vi "FitLinear (SubVI).vi"(0 "Normalized Intensity vs Radius in":cluster{dbl[], dbl[]}, 1 "x values":dbl[](array[numeric]), 2 "y values":dbl[](array[numeric]), 3 "Estimated mean":dbl, 4 "Estimated width":dbl, 6 "parameter bounds":T1={"slope min"=-inf, "slope max"=inf, "intercept min"=-inf, "intercept max"=inf}, 7 "Nsigma Low":dbl=4.0 format="%#_13g", 8 "Use all points":bool, 9 "Nsigma High":dbl=4.0 format="%#_13g") -> (14 "data plot":cluster{dbl[], dbl[]}(graph), 15 "derivative data plot with linear fit":T2(graph), 16 "slope":dbl, 17 "intercept":dbl, 18 "error":i32, 19 "residue":dbl)   [LabVIEW 2016]
uses:
  <vilib>/Analysis/NI_AALPro.lvlib
panel:
  # "RESULTS"
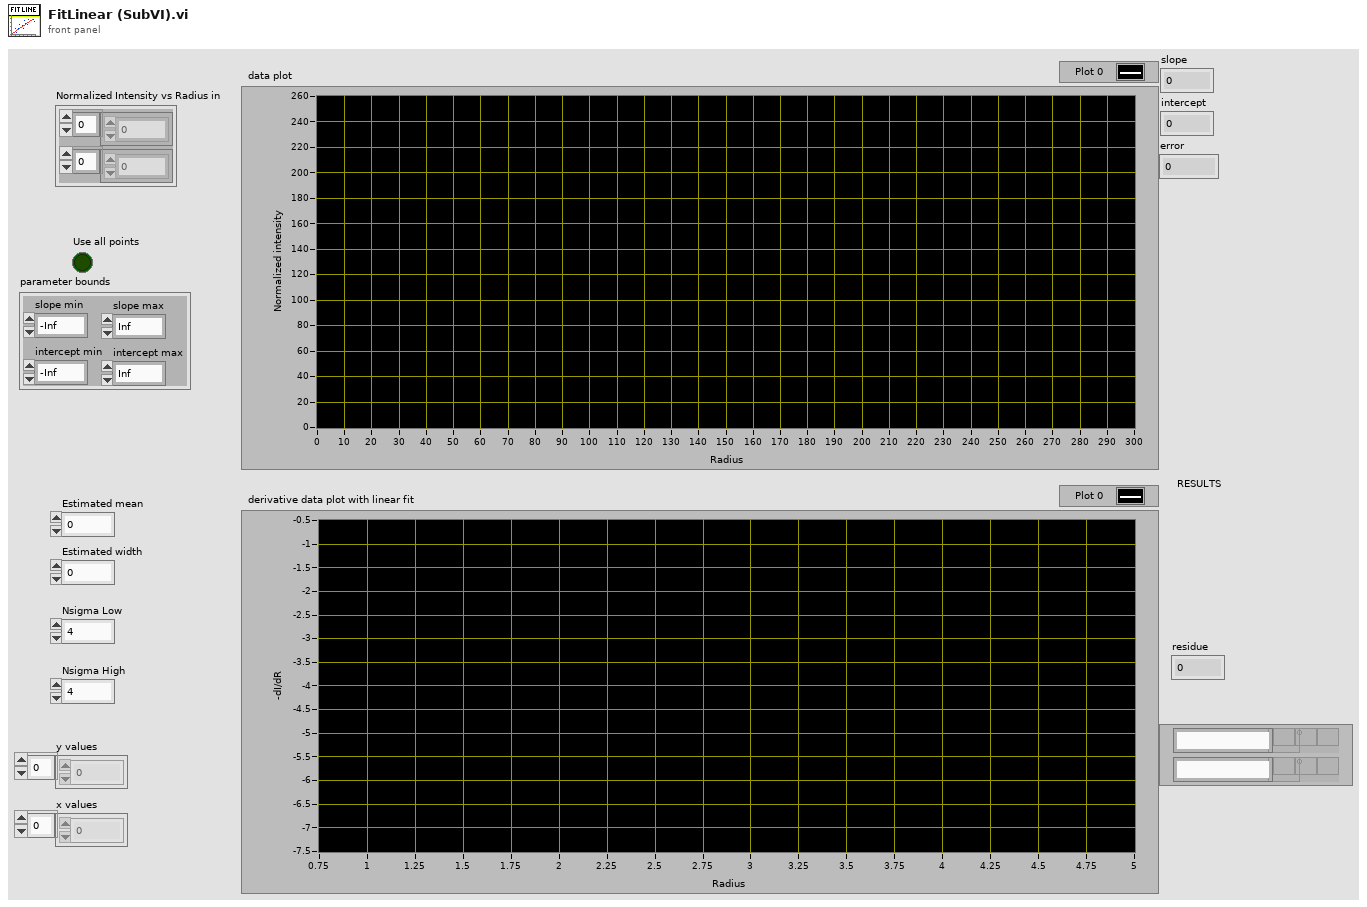
[diagram p1: front panel]
types:
  T1 = cluster{"slope min":dbl, "slope max":dbl, "intercept min":dbl, "intercept max":dbl}
  T2 = cluster{"Radius bins":dbl[], "Best Gaussian Fit":dbl[]}[]
  T3 = cluster{"x values":dbl[], "Best Linear Fit":dbl[]}
  T4 = cluster{"x values":dbl[], "Best Linear Fit":dbl[]}[]
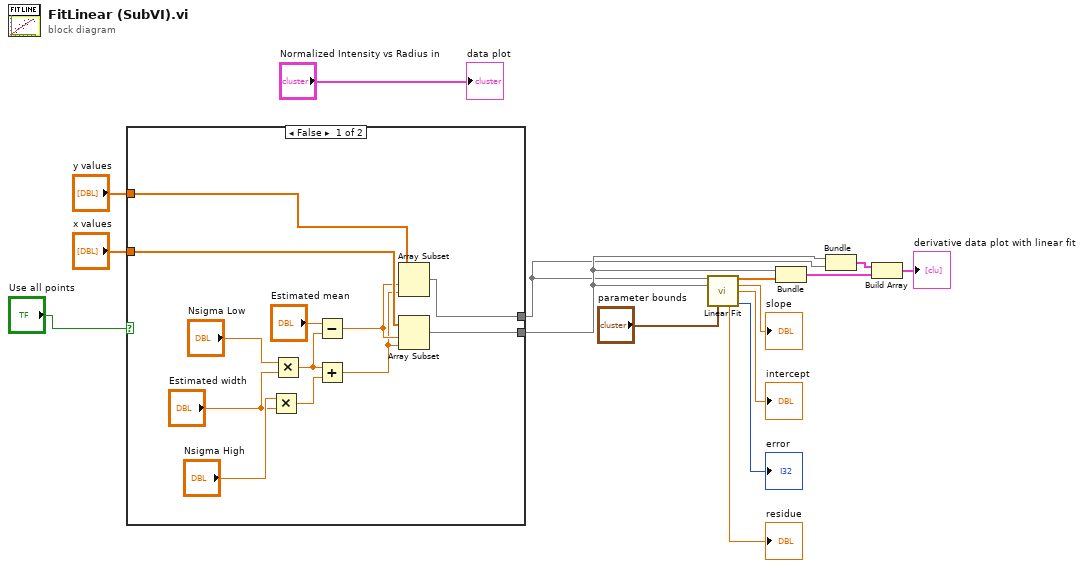
[diagram p0: block diagram]
diagram:
  n1 = case shown="False" "Use all points" {
    tunnel: "y values" -> [w25 w28]
    tunnel: [w24 w28] -> w6
    tunnel: "x values" -> [w23 w29]
    tunnel: [w22 w29] -> w9
    frame False {
      n2 = Multiply(x="Nsigma High", y="Estimated width") -> (x*y=w17:dbl)
      n3 = Multiply(x="Nsigma Low", y="Estimated width") -> (x*y=w18:dbl)
      n4 = Subtract(x="Estimated mean", y=w18) -> (x-y=w21:dbl)
      n5 = Add(x=w18, y=w17) -> (x+y=w16:dbl)
      n6 = Array Subset(array=w25, index=w21, length=w16) -> (w24:dbl[])
      n7 = Array Subset(array=w23, index=w21, length=w16) -> (w22:dbl[])
    }
    frame True {
    }
  }
  n8 = call <vilib>:"Linear Fit.vi"("Y"=w6, "X"=w9, "parameter bounds"="parameter bounds") -> ("Best Linear Fit"=w14:dbl[], "slope"=→"slope":dbl, "intercept"=→"intercept":dbl, "residue"=→"residue":dbl, "error"=→"error":i32)  [unwired: 8 in]
  n9 = Bundle("x values"=w9, "Best Linear Fit"=w14) -> (w13:T3)  [unwired: 1 in]
  n10 = Bundle("x values"=w9, "y values"=w6) -> (w7:cluster{"x values":dbl[], "y values":dbl[]})  [unwired: 1 in]
  n11 = Build Array(w7, w13) -> (→"derivative data plot with linear fit":T4)
  "data plot" <- "Normalized Intensity vs Radius in"
